vi "pololuDriverDIR_v1.vi"(10 "Direction":bool, 11 "Duty Cycle":dbl) -> (2 "PWM 2 Out":fxp<+,32,0>, 3 "PWM 1 Out":fxp<+,32,0>)   [LabVIEW 2016]
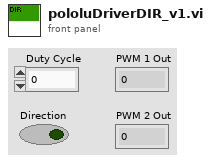
[diagram p1: front panel]
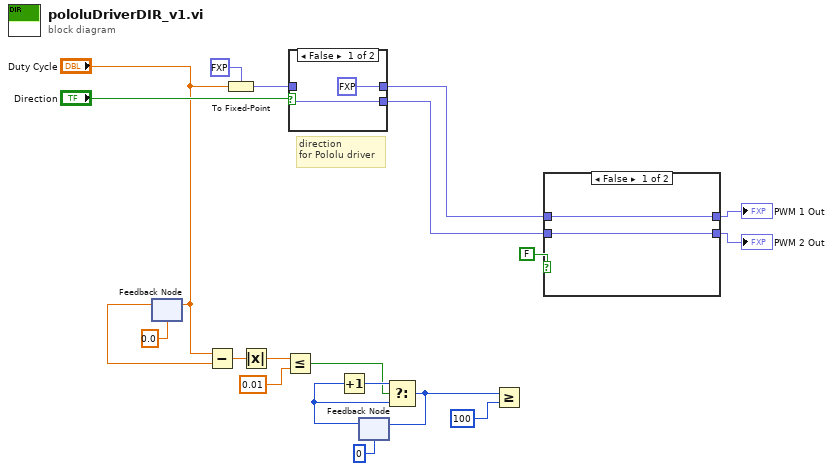
[diagram p0: block diagram]
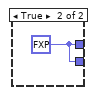
[diagram p2: hidden frame]
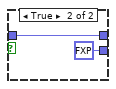
[diagram p3: hidden frame]
diagram:
  # "direction\nfor Pololu driver"
  n1 = feedback-in #1("Duty Cycle") -> ()
  n2 = feedback #1(0.0 ("Duty Cycle")) -> (w15:dbl)
  n3 = Subtract(x="Duty Cycle", y=w15) -> (x-y=w14:dbl)
  n4 = To Fixed-Point(fixed-point type=fxp<+,32,0> 0.0 ("X PWM 2"), number="Duty Cycle") -> (fixed-point=w19:fxp<+,32,0>)
  n5 = Absolute Value(x=w14) -> (abs(x)=w13:dbl)
  n6 = Less Or Equal?(x=w13, y=0.01) -> (x <= y?=w8:bool)
  n7 = case shown="False" "Direction" {
    tunnel: [fxp<+,32,0> 0.0 ("X PWM 2") w24] -> w5
    tunnel: w19 -> [w22 w24]
    tunnel: [w22 fxp<+,32,0> 0.0 ("X PWM 2")] -> w4
    frame False {
    }
    frame True {
    }
  }
  n8 = feedback #2(u16 0 ("Mismatch Tol")) -> (w10:u16)
  n9 = Increment(x=w10) -> (x+1=w9:u16)
  n10 = Select(t=w9, s=w8, f=w10) -> (s? t:f=w7:u16)
  n11 = feedback-in #2(w7) -> ()
  n12 = Greater Or Equal?(x=w7, y=u16 100) -> ()  [unwired: 1 out]
  n13 = case shown="False" FALSE {
    tunnel: w5 -> [w26 _]
    tunnel: w4 -> [w25 _]
    tunnel: [w26 w27] -> w3
    tunnel: [w25 w27] -> w2
    frame False {
    }
    frame True {
      w27 = fxp<+,32,0> 0.0 ("X PWM 2")
    }
  }
  "PWM 2 Out" <- w2
  "PWM 1 Out" <- w3
